vi "Load Client Design.vi"(8 "error in (no error)":errorcluster) -> (0 "error out":errorcluster, 1 "Design Inputs":T1={"Q.Plant"=0.005, "C.AlumDoseMax"=0.01, "C.AlumStock"=0.015, "Ti.AlumStock"=0.0015, "EN.DrillSeries"=enum."English", "EN.TubeSeries"=enum."English", "EN.PipeSeries"=enum."SDR 41\n", "N.SedTanks"=240.0, "N.SedBaysEst"=2.0, "W.SedPlate"=0.0, "L.SedPlateSheet"=388800000.0, "T.SedPlate"=0.03, "T.PlantWall"=0.01, "H.FlocOption"=0.03, "T.FlocBaffleRigidH"=0.3, "T.ConcreteMin"=0.3, "T.SedWeir"=108000.0, "T.FlocBaffleRigidV"=0.04} {"T.FlocBaffleRigidV" min=0.0 max=0.2 step=0.001 format="%#.1f"; "T.SedWeir" min=0.001 max=0.2 step=0.001 format="%#.1f"; "T.SedPlate" min=0.001 max=0.05 step=0.001 format="%#.1f"; "T.FlocBaffleRigidH" min=0.0 max=0.2 step=0.001 format="%#.1f"; "T.ConcreteMin" min=0.005 max=0.2 step=0.001 format="%#.1f"; "L.SedPlateSheet" min=0.3 max=8.0 step=0.01 format="%#.1f"; "N.SedBaysEst" min=1.0 max=20.0 step=1.0 format="%#.0f"; "N.SedTanks" min=1.0 max=20.0 step=1.0 format="%#.0f"; "Ti.AlumStock" min=43200.0 max=360000.0 step=3600.0 format="%#.1f"; "H.FlocOption" min=0.5 max=4.0 step=0.01 format="%#.2f"; "C.AlumStock" min=50.0 max=500.0 step=1.0 format="%#.0f"; "C.AlumDoseMax" min=0.03 max=0.2 step=0.005 format="%#.0f"; "Q.Plant" min=0.001 max=0.2 step=0.0001 format="%#.1f"; "T.PlantWall" min=0.05 max=0.5 step=0.001 format="%#.1f"; "W.SedPlate" min=0.5 max=3.0 step=0.001 format="%#.1f"}, 2 "Project Info":T2)   [LabVIEW 2010]
uses:
  Project inputs.ctl
  Basic Inputs.ctl
  Instance           1 26Saved   Load Client Design .vi
  AguaClara Library.lvlib
panel:
  out "data":cluster{"Label.Text":string, "Value":variant}[](array[cluster])
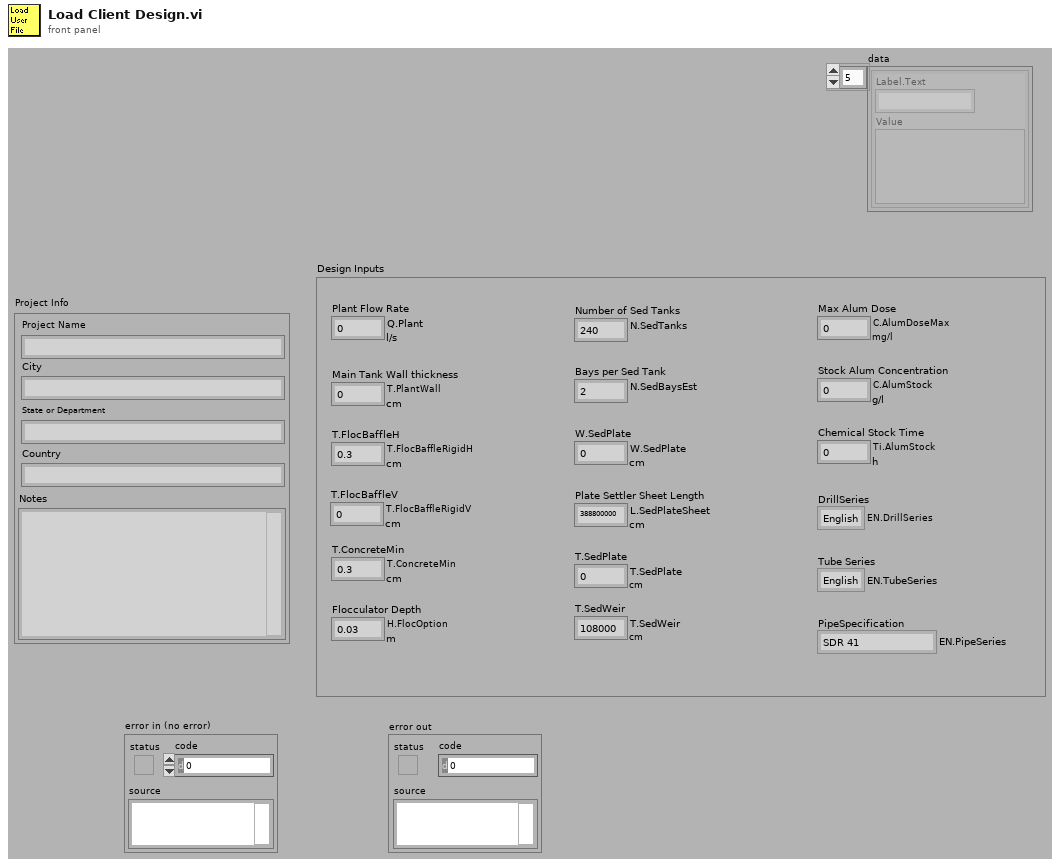
[diagram p1: front panel]
types:
  T1 = typedef "AguaClara Library.lvlib/Basic Inputs.ctl" = cluster{"Q.Plant":dbl[unit], "C.AlumDoseMax":dbl[unit], "C.AlumStock":dbl[unit], "Ti.AlumStock":dbl[unit], "EN.DrillSeries":enum16{"English", "Metric"}, "EN.TubeSeries":enum16{"English", "Metric"}, "EN.PipeSeries":enum16{"Schedule Number 10", "Schedule number 30\n", "Schedule Number 40", "Schedule Number 80\n", "Schedule Number 120", "Schedule Number 160\n", "SDR 17\n", "SDR 21\n", "SDR 26\n", "SDR 32.5\n", "SDR 41\n"}, "N.SedTanks":dbl, "N.SedBaysEst":dbl, "W.SedPlate":dbl[unit], "L.SedPlateSheet":dbl[unit], "T.SedPlate":dbl[unit], "T.PlantWall":dbl[unit], "H.FlocOption":dbl[unit], "T.FlocBaffleRigidH":dbl[unit], "T.ConcreteMin":dbl[unit], "T.SedWeir":dbl[unit], "T.FlocBaffleRigidV":dbl[unit]}
  T2 = typedef "AguaClara Library.lvlib/Project inputs.ctl" = cluster{"Project Name":string, "City":string, "State":string, "Country":string, "Notes":string}
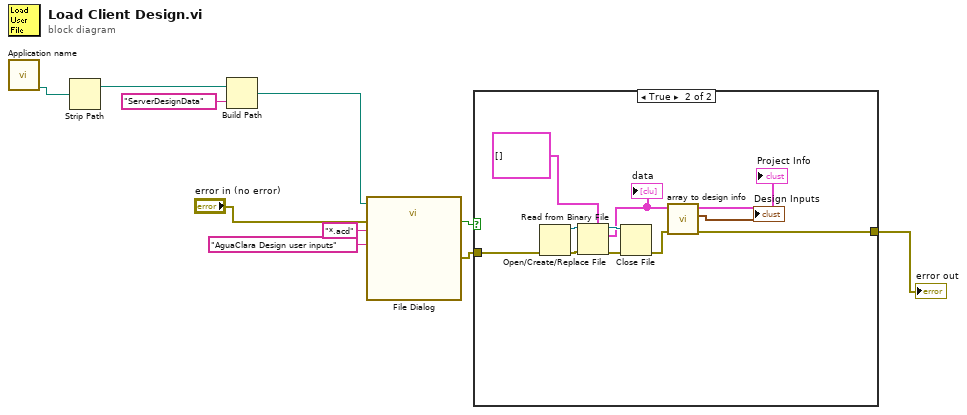
[diagram p0: block diagram]
diagram:
  n1 = call "Application name.vi"() -> ("Ini file path"=w4:path)  [unwired: 4 in, 3 out]
  n2 = Strip Path(path=w4) -> (stripped path=w3:path)  [unwired: 1 out]
  n3 = Build Path(base path=w3, name or relative path="ServerDesignData") -> (appended path=w1:path)
  n4 = call "File Dialog"("start path"=w1, "error in"="error in (no error)", "pattern (all files)"="*.acd", "pattern label"="AguaClara Design user inputs") -> ("exists"=w8:bool, "error out"=w9:errorcluster)  [unwired: 8 in, 2 out]
  n5 = case shown="True" w8 {
    tunnel: w9 -> [w11 w13]
    tunnel: [w11 w12] -> w7
    frame False {
    }
    frame True {
      n6 = Open/Create/Replace File(error in=w13) -> (refnum out=w22:refnum<file>, error out=w19:errorcluster)  [unwired: 5 in, 1 out]
      n7 = Read from Binary File(5:cluster{"Label.Text":string, "Value":variant}[] [] ("data"), 8:w19, 11:w22) -> (0:w20:errorcluster, 2:w18:cluster{"Label.Text":string, "Value":variant}[], 3:w21:refnum<file>)  [unwired: 3 in, 1 out]
      "data" <- w18
      n8 = Close File(refnum=w21, error in=w20) -> (error out=w15:errorcluster)  [unwired: 1 out]
      n9 = call "array to design info.vi"("error in (no error)"=w15, "Array from file"=w18) -> ("error out"=w12:errorcluster, "Design Inputs"=→"Design Inputs":T1, "Project Info"=→"Project Info":T2)  [unwired: 7 in]
    }
  }
  "error out" <- w7
